vi "OxITC503 _Config_ Setpoint.vi"(2 "error in":errorcluster, 3 "Setpoint":dbl format="%.2f", 4 "VISA session":refnum<visa-resource-name>) -> (0 "error out (no error)":errorcluster, 1 "VISA session":refnum<visa-resource-name>)   [LabVIEW 2014]
doc: "Sets a set point temperature."
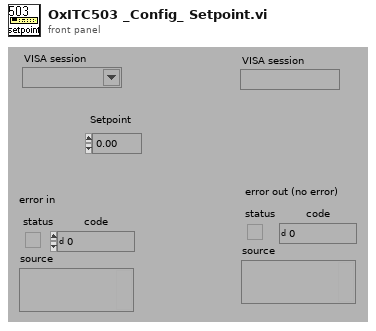
[diagram p1: front panel]
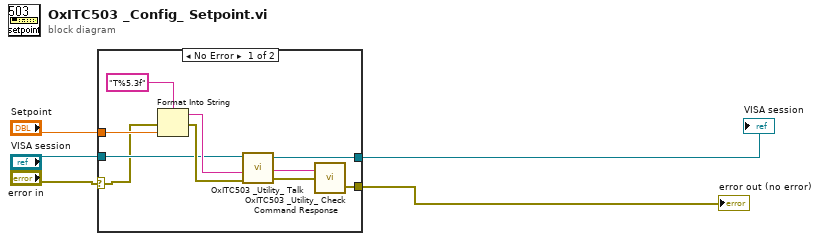
[diagram p0: block diagram]
diagram:
  n1 = case shown="No Error" "error in" {
    selector: "error in" -> [w6 w16]
    tunnel: "Setpoint" -> [w13 _]
    tunnel: [w11 w17] -> w4
    tunnel: "VISA session" -> [w10 w17]
    tunnel: [w7 w16] -> w2
    frame No Error {
      n2 = Format Into String(format string="T%5.3f" ("Format String"), error in=w6, w13) -> (resulting string=w14:string, error out=w15:errorcluster)  [unwired: 1 in]
      n3 = call "OxITC503 _Utility_ Talk.vi"("VISA session"=w10, "Command"=w14, "error in (no error)"=w15) -> ("VISA session"=w11:refnum<visa-resource-name>, "read buffer"=w8:string, "error out (no error)"=w9:errorcluster)  [unwired: 2 in]
      n4 = call "OxITC503 _Utility_ Check Command Response.vi"("error in"=w9, "read buffer"=w8) -> ("error out (no error)"=w7:errorcluster)  [unwired: 1 out]
    }
    frame Error {
    }
  }
  "error out (no error)" <- w2
  "VISA session" <- w4
